vi "Execute AT command.vi"(5 "Exit AT mode":bool, 6 "milliseconds to wait":u32=100, 7 "error in (no error)":errorcluster, 8 "AT Command":string, 10 "VISA resource in":refnum<visa-resource-name>) -> (0 "error out":errorcluster, 2 "Response message":string, 3 "VISA resource out":refnum<visa-resource-name>)   [LabVIEW 2016]
uses:
  <vilib>/Instr/_visa.llb/VISA Flush IO Buffer Mask.ctl
  Mode enum.ctl
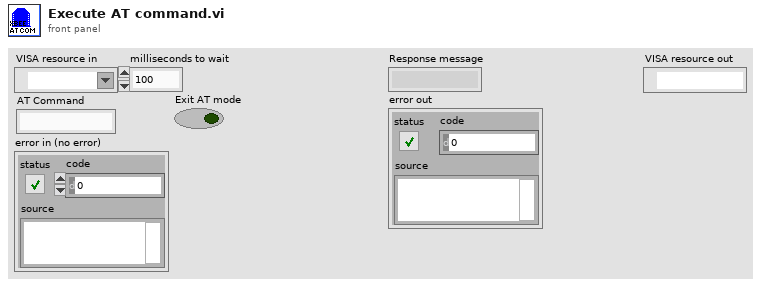
[diagram p1: front panel]
types:
  T1 = typedef "Mode enum.ctl" = enum16{"Other", "Command mode"}
  T2 = typedef "VISA Flush IO Buffer Mask.ctl" = u16
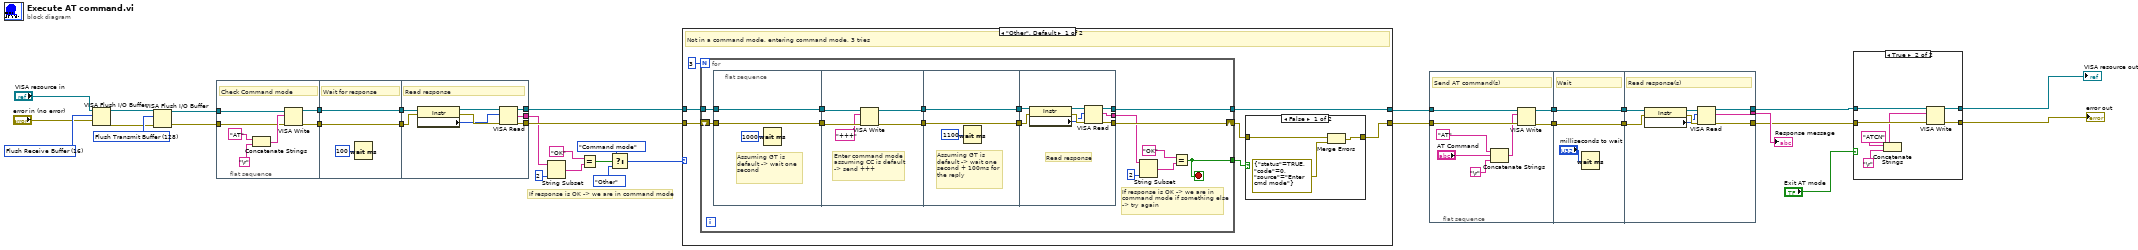
[diagram p0: block diagram]
diagram:
  w29 = T2 16 items=["Flush Receive Buffer"=16, "Write Transmit Buffer to Device"=32, "Flush Receive Buffer (No I/O)"=64, "Flush Transmit Buffer"=128] ("Mask")
  w34 = T2 128 items=["Flush Receive Buffer"=16, "Write Transmit Buffer to Device"=32, "Flush Receive Buffer (No I/O)"=64, "Flush Transmit Buffer"=128] ("Mask")
  # "If response is OK -> we are in command mode"
  n1 = VISA Flush I/O Buffer(VISA resource name="VISA resource in", mask (16)=w29, error in (no error)="error in (no error)") -> (VISA resource name out=w31:refnum<visa-resource-name>, error out=w30:errorcluster)
  n2 = VISA Flush I/O Buffer(VISA resource name=w31, mask (16)=w34, error in (no error)=w30) -> (VISA resource name out=w33:refnum<visa-resource-name>, error out=w32:errorcluster)
  n3 = flat-sequence {
    tunnel: w33 -> [w41]
    tunnel: w32 -> [w38]
    tunnel: [w36] -> w11
    tunnel: [w35] -> w10
    tunnel: w11 -> [w43]
    tunnel: w10 -> [w42]
    tunnel: [w43] -> w9
    tunnel: [w42] -> w8
    tunnel: w9 -> [w52]
    tunnel: w8 -> [w51]
    tunnel: [w47] -> w26
    tunnel: [w46] -> w25
    tunnel: [w45] -> w7
    frame #0 {
      # "Check Command mode"
      n4 = Concatenate Strings("AT" ("string"), "\r") -> (w39:string)
      n5 = VISA Write(VISA resource name=w41, write buffer=w39, error in (no error)=w38) -> (VISA resource name out=w36:refnum<visa-resource-name>, error out=w35:errorcluster)  [unwired: 1 out]
    }
    frame #1 {
      # "Wait for response"
      n6 = Wait (ms)(milliseconds to wait=u32 100 ("millisecond multiple")) -> ()  [unwired: 1 out]
    }
    frame #2 {
      # "Read response"
      n7 = property class="Instr"(reference=w52, error in=w51) -> (reference out=w50:refnum<visa-resource-name>, error out=w49:errorcluster, "Serial Settings:Number of Bytes at Serial Port"=w48:u32)
      n8 = VISA Read(VISA resource name=w50, byte count=w48, error in (no error)=w49) -> (VISA resource name out=w47:refnum<visa-resource-name>, read buffer=w45:string, error out=w46:errorcluster)  [unwired: 1 out]
    }
  }
  n9 = String Subset(string=w7, length (rest)=2 ("length (rest)")) -> (substring=w5:string)  [unwired: 1 in]
  n10 = Equal?(x="OK", y=w5) -> (x = y?=w3:bool)
  n11 = Select(t=Mode_enum."Command mode", s=w3, f=Mode_enum."Other") -> (s? t:f=w27:T1)
  n12 = case shown="\"Other\", Default" w27 {
    tunnel: w26 -> [w59 w99]
    tunnel: w25 -> [w58 w98]
    tunnel: [w57 w99] -> w24
    tunnel: [w53 w98] -> w23
    frame "Other", Default {
      # "Not in a command mode, entering command mode, 3 tries"
      n13 = for {
        N: 3 -> [_]
        shift-right: [w69] -> w54
        shift-left: w58 -> [w71]
        tunnel: w59 -> [w72]
        tunnel: [w70] -> w57
        tunnel: [w64] -> w55
        stop <- w64 stop-if-true
        # "If response is OK -> we are in command mode if something else -> try again"
        n14 = flat-sequence {
          tunnel: w72 -> [w80]
          tunnel: w71 -> [w79]
          tunnel: [w80] -> w78
          tunnel: [w79] -> w77
          tunnel: w78 -> [w86]
          tunnel: w77 -> [w85]
          tunnel: [w84] -> w76
          tunnel: [w83] -> w75
          tunnel: w76 -> [w89]
          tunnel: w75 -> [w88]
          tunnel: [w89] -> w74
          tunnel: [w88] -> w73
          tunnel: [w91] -> w69
          tunnel: [w92] -> w70
          tunnel: w74 -> [w97]
          tunnel: w73 -> [w96]
          tunnel: [w90] -> w65
          frame #0 {
            # "Assuming GT is default -> wait one second"
            n15 = Wait (ms)(milliseconds to wait=u32 1000) -> ()  [unwired: 1 out]
          }
          frame #1 {
            # "Enter command mode assuming CC is default -> send +++"
            n16 = VISA Write(VISA resource name=w86, write buffer="+++", error in (no error)=w85) -> (VISA resource name out=w84:refnum<visa-resource-name>, error out=w83:errorcluster)  [unwired: 1 out]
          }
          frame #2 {
            # "Assuming GT is default -> wait one second + 100ms for the reply"
            n17 = Wait (ms)(milliseconds to wait=u32 1100) -> ()  [unwired: 1 out]
          }
          frame #3 {
            # "Read response"
            n18 = property class="Instr"(reference=w97, error in=w96) -> (reference out=w93:refnum<visa-resource-name>, error out=w95:errorcluster, "Serial Settings:Number of Bytes at Serial Port"=w94:u32)
            n19 = VISA Read(VISA resource name=w93, byte count=w94, error in (no error)=w95) -> (VISA resource name out=w92:refnum<visa-resource-name>, read buffer=w90:string, error out=w91:errorcluster)  [unwired: 1 out]
          }
        }
        n20 = String Subset(string=w65, length (rest)=2 ("length (rest)")) -> (substring=w67:string)  [unwired: 1 in]
        n21 = Equal?(x="OK", y=w67) -> (x = y?=w64:bool)
      }
      n22 = case shown="False" w55 {
        tunnel: w54 -> [w61 w63]
        tunnel: [w62 w63] -> w53
        frame False {
          n23 = Merge Errors(w61, errorcluster {"status"=TRUE, "code"=0, "source"="Enter cmd mode"} ("error constant")) -> (w62:errorcluster)
        }
        frame True {
        }
      }
    }
    frame "Command mode" {
      # "In command mode, no action required"
    }
  }
  n24 = flat-sequence {
    tunnel: w24 -> [w107]
    tunnel: w23 -> [w106]
    tunnel: [w101] -> w22
    tunnel: [w100] -> w21
    tunnel: w22 -> [w110]
    tunnel: w21 -> [w109]
    tunnel: [w110] -> w20
    tunnel: [w109] -> w19
    tunnel: w20 -> [w118]
    tunnel: w19 -> [w117]
    tunnel: [w113] -> w18
    tunnel: [w112] -> w14
    tunnel: [w111] -> w15
    frame #0 {
      # "Send AT command(s)"
      n25 = Concatenate Strings("AT" ("string"), "AT Command", "\r") -> (w105:string)
      n26 = VISA Write(VISA resource name=w107, write buffer=w105, error in (no error)=w106) -> (VISA resource name out=w101:refnum<visa-resource-name>, error out=w100:errorcluster)  [unwired: 1 out]
    }
    frame #1 {
      # "Wait"
      n27 = Wait (ms)(milliseconds to wait="milliseconds to wait") -> ()  [unwired: 1 out]
    }
    frame #2 {
      # "Read response(s)"
      n28 = property class="Instr"(reference=w118, error in=w117) -> (reference out=w114:refnum<visa-resource-name>, error out=w116:errorcluster, "Serial Settings:Number of Bytes at Serial Port"=w115:u32)
      n29 = VISA Read(VISA resource name=w114, byte count=w115, error in (no error)=w116) -> (VISA resource name out=w111:refnum<visa-resource-name>, read buffer=w113:string, error out=w112:errorcluster)  [unwired: 1 out]
    }
  }
  n30 = case shown="True" "Exit AT mode" {
    tunnel: w15 -> [w120 w127]
    tunnel: w14 -> [w119 w126]
    tunnel: [w120 w122] -> w13
    tunnel: [w119 w121] -> w12
    frame False {
    }
    frame True {
      n31 = Concatenate Strings("ATCN" ("write buffer"), "\r") -> (w124:string)
      n32 = VISA Write(VISA resource name=w127, write buffer=w124, error in (no error)=w126) -> (VISA resource name out=w122:refnum<visa-resource-name>, error out=w121:errorcluster)  [unwired: 1 out]
    }
  }
  "VISA resource out" <- w13
  "error out" <- w12
  "Response message" <- w18
